vi "Error.Message.Format.vi"(0 "Source":string="Error 333 occurred at source of error", 2 "Details":string="reason for problem\nasdfasdf\tasdfaa sdfja ;sldjf;alskdjf;a lksjdf there is way more to this than meets the eye at first glance ;laiwje;fliajsd;flk ajsdlkfja psoieur a;lwdjf; alksjdf;alksdjf; alksedrfap oiwejf;alkw\nwerasdf\t3425 a b c d e f g h i j k l m n o p q\nafsdfasdfasdfasdfas asdf asdf\tasdfasd") -> (1 "message":string="OK", 5 "Bold Start":i32[](array[numeric]), 6 "Bold Length":i32[](array[numeric]), 7 "Source Out":string="Error 333 occurred at source of error", 8 "Details Out":string)   [LabVIEW 2027, in "VS Inline Async API.lvlib"]
uses:
  VS Inline Async API.lvlib
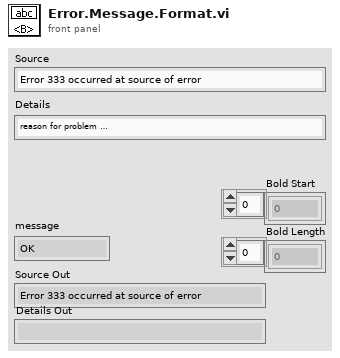
[diagram p1: front panel]
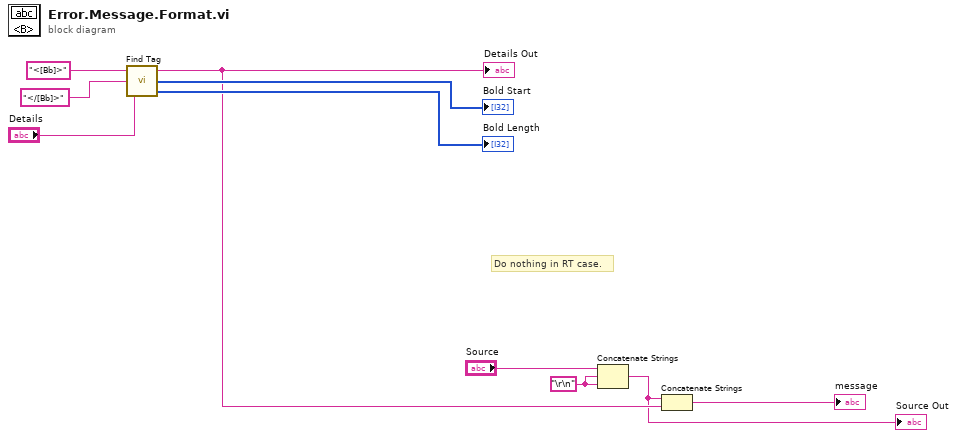
[diagram p0: block diagram]
diagram:
  w8 = "\r\n"
  # "Do nothing in RT case."
  n1 = call <vilib>:"Find Tag.vi"("string"="Details", "close tag"="</[Bb]>" ("don't translate!"), "open tag"="<[Bb]>" ("don't translate!")) -> ("Length"=→"Bold Length":i32[], "Start"=→"Bold Start":i32[], "string out"=w5:string)
  "Details Out" <- w5
  n2 = Concatenate Strings("Source", w8, w8) -> (w3:string)
  "Source Out" <- w3
  n3 = Concatenate Strings(w3, w5) -> (→"message":string)
